vi "Execute SQL.vi"(8 "error in (no error)":errorcluster, 10 "SQL string":string, 11 "Database Viewer":refnum<class "Database Viewer.lvclass">) -> (0 "error out":errorcluster, 2 "SQL Result":string[][](array[string]), 3 "Database Viewer out":refnum<class "Database Viewer.lvclass">)   [LabVIEW 2019, in "Database Viewer.lvclass"]
uses:
  Database Viewer.lvclass
  Database Viewer.lvclass/Database Viewer.ctl
  <userlib>/LevyLab/LV-Data/LV-Data.PG/LV-Data.PGSQL.lvclass
panel:
  out "size(s)":i32[](array[numeric])
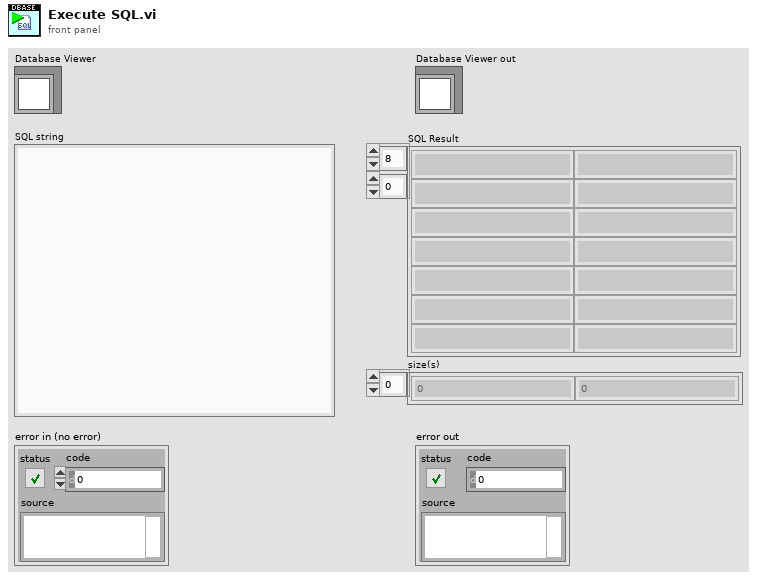
[diagram p1: front panel]
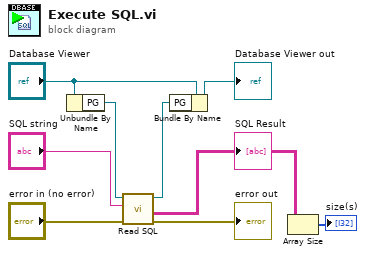
[diagram p0: block diagram]
diagram:
  n1 = Unbundle By Name("Database Viewer") -> ("PG"=w3:refnum<class "LV-Data.PGSQL.lvclass">)
  n2 = call <userlib>:"Read SQL.vi"("error in (no error)"="error in (no error)", "SQL string"="SQL string", "Data.PGQL in"=w3) -> ("error out"=→"error out":errorcluster, "Result"=w2:string[][], "Data.PGSQL out"=w5:refnum<class "LV-Data.PGSQL.lvclass">)  [unwired: 5 in, 1 out]
  "SQL Result" <- w2
  n3 = Bundle By Name(cluster="Database Viewer", "PG"=w5) -> (→"Database Viewer out":refnum<class "Database Viewer.lvclass">)
  n4 = Array Size(array=w2) -> (size(s)=→"size(s)":i32[])
